vi "DCAM_show_preview_update_camera.vi"() -> ()   [LabVIEW 2015]
panel:
  out "S Start Trig Mode":dbl
  out "S Binning":dbl
  in  "Start Trigger Mode":u32(ring)=1 items=["Internal"=1, "External Edge"=2, "External Level"=4, "Software"=32, "Fast Repetition"=64, "TDI"=128, "Trigger Start"=512, "Sync Readout"=1024]
  in  "Binning":u16(ring) items=["1x1"=1, "2x2"=2, "4x4"=4]
  out "S Vert Offset":i32
  out "S Horiz Offset":i32
  in  "Vertical Offset":i32 min=0 max=0 step=4
  in  "Horizontal Offset":i32 min=0 max=0 step=4
  in  "Scan Mode":dbl min=1.0 max=2.0 step=1.0
  out "S Scan Mode":dbl min=1.0 max=2.0 step=1.0
  in  "Exposure":dbl min=0.0010036691729323308 max=10.000004210526315 step=1e-08
  out "S Exposure":dbl
  out "S Vert Width":i32
  out "S Horiz Width":i32
  in  "Vertical Width":i32 min=4 max=2048 step=4
  in  "Horizontal Width":i32 min=4 max=2048 step=4
  out "error out":errorcluster
  out "DCAM Ver.":string
  out "Library Ver.":string
  out "Firmware":string
  out "Camera ID":string
  out "Model":string
  out "Timeseries Base Filename":string
  out "Timeseries Save Path":path
  in  "Start Button":bool
  out "Image":u16[][](graph)
  in  "Stop":bool
  out "Frames Recorded":i32
  in  "Frames":i32=100
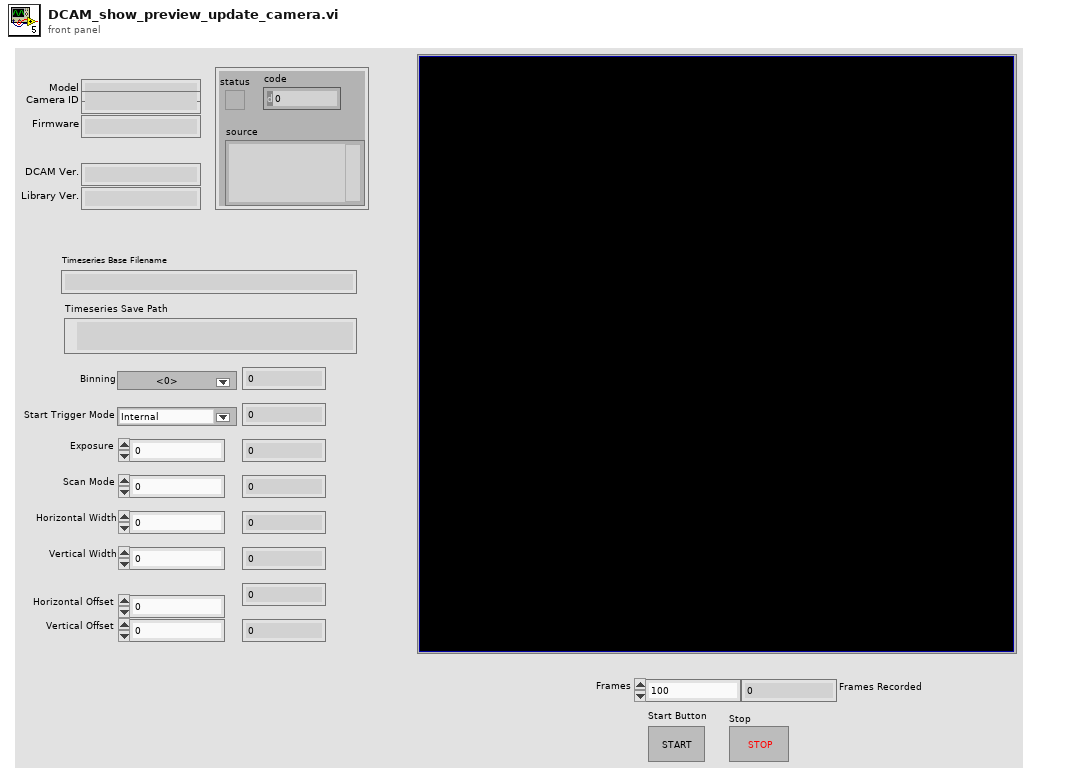
[diagram p1: front panel]
types:
  T1 = cluster{"Capture Library":string, "DCAM-API":string}
  T2 = cluster{"Model":string, "Camera ID":string, "Firmware":string}
  T3 = cluster{"Value":i32, "Minimum":i32, "Maximum":i32, "Increment":i32}
  T4 = cluster{"height":u32, "width":u32, "datatype":u32}
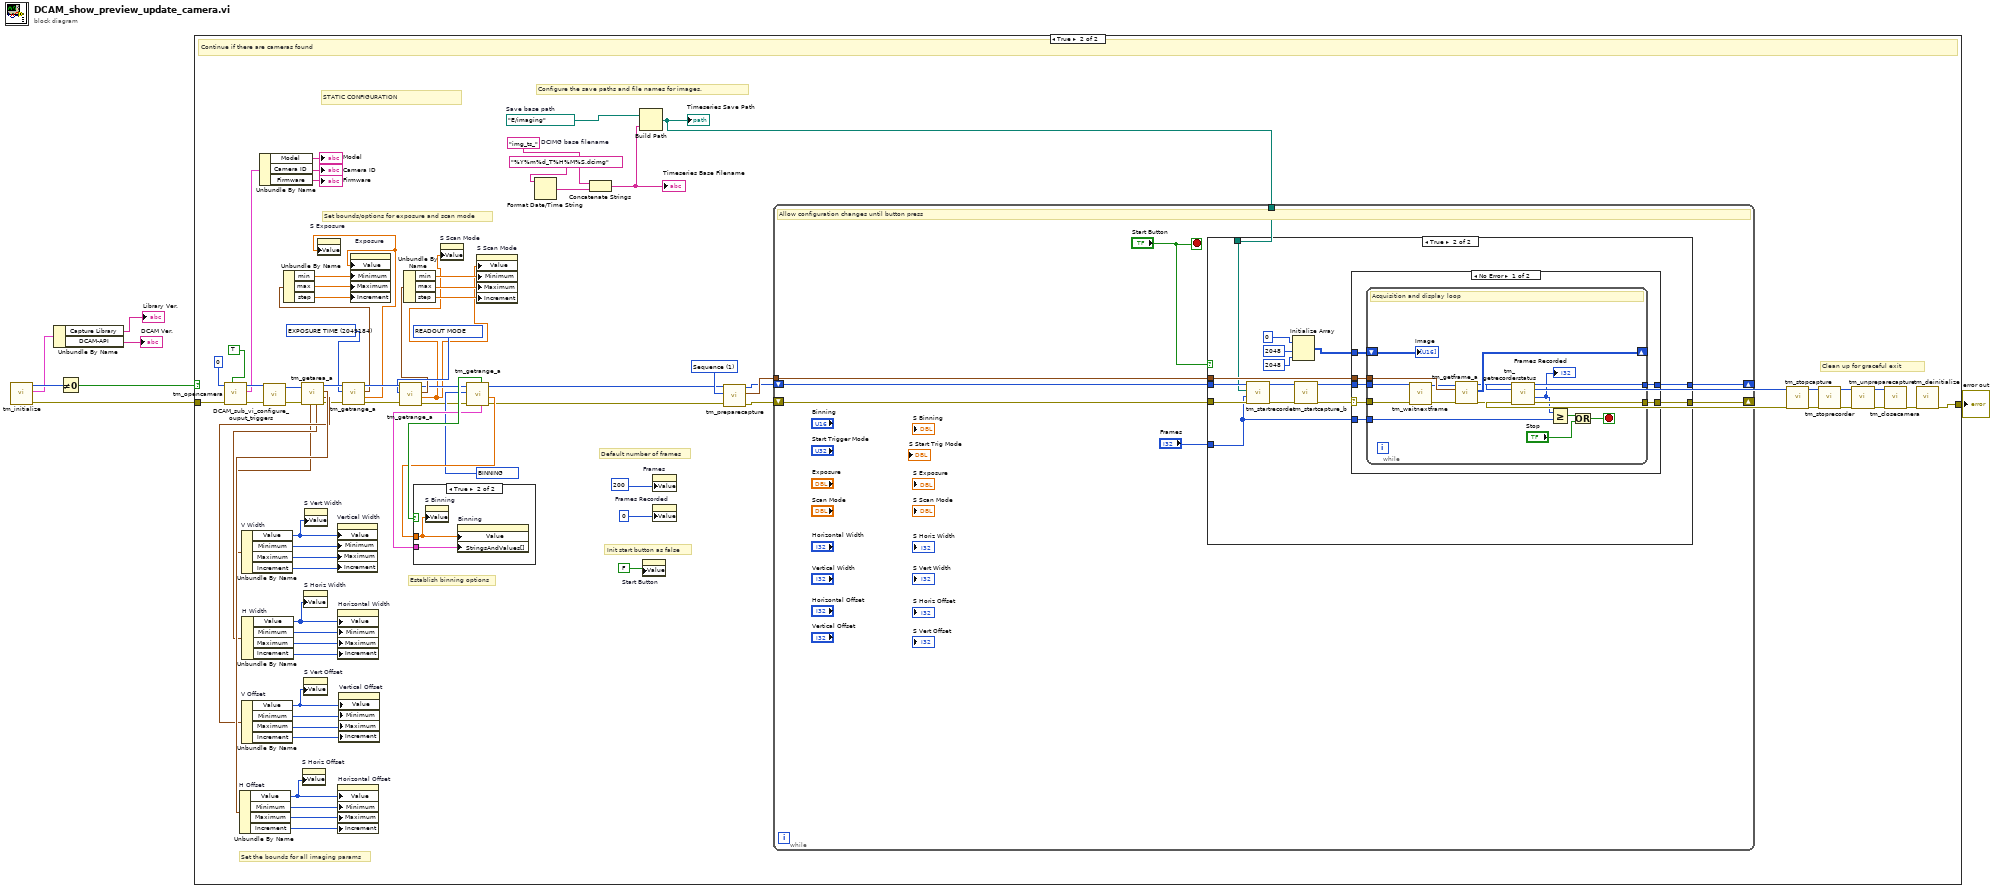
[diagram p0: block diagram]
diagram:
  n1 = call <userlib>:"tm_initialize.vi"() -> ("error out"=w2:errorcluster, "Version Info"=w5:T1, "Number Of Cameras"=w7:u32)  [unwired: 8 in, 1 out]
  n2 = Unbundle By Name(w5) -> ("Capture Library"=→"Library Ver.":string, "DCAM-API"=→"DCAM Ver.":string)
  n3 = Not Equal To 0?(x=w7) -> (x != 0?=w6:bool)
  n4 = case shown="True" w6 {
    tunnel: w2 -> [w8 w85]
    tunnel: [w8 w74] -> w1
    frame False {
    }
    frame True {
      w15 = u32 4215968 items=["BINNING"=4215968, "BITS PER CHANNEL"=4342976, "ACTIVE VIEW INDEX"=4343136, "CCD MODE"=4212384, "SENSOR MODE"=4212128, "READOUT MODE"=4211872, "EXPOSURE TIME"=2049184, "CONTRAST GAIN"=3163312, "CONTRAST OFFSET"=3163328, "LIGHT MODE"=2114720, "SENSITIVITY"=2114992, "WHITE BALANCE"=3163568, "PHOTON IMAGING MODE"=2115200, "HIGH DYNAMIC RANGE MODE"=3163360, "TRIGGER SOURCE"=1066144, "TRIGGER ACTIVE"=1066160, "TRIGGER MODE"=1066400, "TRIGGER POLARITY"=1066416, "TRIGGER GLOBAL EXPOSURE"=2049680, "FIRST TRIGGER BEHAVIOR"=2049696, "TRIGGER TIMES"=1066448, "OUTPUT TRIGGER POLARITY"=1852592, "OUTPUT TRIGGER DELAY"=1852624, "OUTPUT TRIGGER PERIOD"=1852640, "TEMPERATURE"=2115232, "TEMPERATURE TARGET"=2115264, "SENSOR COOLER FAN"=2115296, "MECHANICAL SHUTTER"=2115488, "BACK FOCUS POSITION"=8422304, "FRAMEBUNDLE MODE"=4346784, "FRAMEBUNDLE NUMBER"=4346800, "LINEBUNDLE HEIGHT"=4212192, "TRIGGER CONNECTOR"=1066432, "IMAGE PIXEL TYPE"=4343296, "OUTPUT TRIGGER KIND"=1852656, "READOUT DIRECTION"=4211904, "CHANNEL SYNC"=1852352] ("Parameter")
      w21 = u32 4211872 items=["BINNING"=4215968, "BITS PER CHANNEL"=4342976, "ACTIVE VIEW INDEX"=4343136, "CCD MODE"=4212384, "SENSOR MODE"=4212128, "READOUT MODE"=4211872, "EXPOSURE TIME"=2049184, "CONTRAST GAIN"=3163312, "CONTRAST OFFSET"=3163328, "LIGHT MODE"=2114720, "SENSITIVITY"=2114992, "WHITE BALANCE"=3163568, "PHOTON IMAGING MODE"=2115200, "HIGH DYNAMIC RANGE MODE"=3163360, "TRIGGER SOURCE"=1066144, "TRIGGER ACTIVE"=1066160, "TRIGGER MODE"=1066400, "TRIGGER POLARITY"=1066416, "TRIGGER GLOBAL EXPOSURE"=2049680, "FIRST TRIGGER BEHAVIOR"=2049696, "TRIGGER TIMES"=1066448, "OUTPUT TRIGGER POLARITY"=1852592, "OUTPUT TRIGGER DELAY"=1852624, "OUTPUT TRIGGER PERIOD"=1852640, "TEMPERATURE"=2115232, "TEMPERATURE TARGET"=2115264, "SENSOR COOLER FAN"=2115296, "MECHANICAL SHUTTER"=2115488, "BACK FOCUS POSITION"=8422304, "FRAMEBUNDLE MODE"=4346784, "FRAMEBUNDLE NUMBER"=4346800, "LINEBUNDLE HEIGHT"=4212192, "TRIGGER CONNECTOR"=1066432, "IMAGE PIXEL TYPE"=4343296, "OUTPUT TRIGGER KIND"=1852656, "READOUT DIRECTION"=4211904, "CHANNEL SYNC"=1852352] ("Parameter")
      w26 = u32 2049184 items=["BINNING"=4215968, "BITS PER CHANNEL"=4342976, "ACTIVE VIEW INDEX"=4343136, "CCD MODE"=4212384, "SENSOR MODE"=4212128, "READOUT MODE"=4211872, "EXPOSURE TIME"=2049184, "CONTRAST GAIN"=3163312, "CONTRAST OFFSET"=3163328, "LIGHT MODE"=2114720, "SENSITIVITY"=2114992, "WHITE BALANCE"=3163568, "PHOTON IMAGING MODE"=2115200, "HIGH DYNAMIC RANGE MODE"=3163360, "TRIGGER SOURCE"=1066144, "TRIGGER ACTIVE"=1066160, "TRIGGER MODE"=1066400, "TRIGGER POLARITY"=1066416, "TRIGGER GLOBAL EXPOSURE"=2049680, "FIRST TRIGGER BEHAVIOR"=2049696, "TRIGGER TIMES"=1066448, "OUTPUT TRIGGER POLARITY"=1852592, "OUTPUT TRIGGER DELAY"=1852624, "OUTPUT TRIGGER PERIOD"=1852640, "TEMPERATURE"=2115232, "TEMPERATURE TARGET"=2115264, "SENSOR COOLER FAN"=2115296, "MECHANICAL SHUTTER"=2115488, "BACK FOCUS POSITION"=8422304, "FRAMEBUNDLE MODE"=4346784, "FRAMEBUNDLE NUMBER"=4346800, "LINEBUNDLE HEIGHT"=4212192, "TRIGGER CONNECTOR"=1066432, "IMAGE PIXEL TYPE"=4343296, "OUTPUT TRIGGER KIND"=1852656, "READOUT DIRECTION"=4211904, "CHANNEL SYNC"=1852352] ("Parameter")
      w73 = 1 items=["Snap", "Sequence"] ("Capture mode")
      w59 = "img_ts_"  # DCIMG base filename
      w62 = path "E:/imaging"  # Save base path
      # "STATIC CONFIGURATION"
      # "Set bounds/options for exposure and scan mode"
      # "Establish binning options"
      # "Set the bounds for all imaging params"
      # "Init start button as false"
      # "Clean up for graceful exit"
      # "Default number of frames"
      # "Configure the save paths and file names for images."
      # "Continue if there are cameras found"
      n5 = call <userlib>:"tm_opencamera.vi"("Force Open"=TRUE, "error in (no error)"=w85, "Camera Index"=0) -> ("error out"=w82:errorcluster, "Camera Details"=w78:T2, "Handle out"=w83:u32)  [unwired: 6 in]
      n6 = Unbundle By Name(w78) -> ("Model"=→"Model":string, "Camera ID"=→"Camera ID":string, "Firmware"=→"Firmware":string)
      n7 = call "DCAM_sub_vi_configure_ouput_triggers.vi"("error in (no error)"=w82, "Handle in"=w83) -> ("error out"=w41:errorcluster, "Handle out"=w42:u32)  [unwired: 2 in]
      n8 = call <userlib>:"tm_getarea_a.vi"("error in (no error)"=w41, "Handle in"=w42) -> ("error out"=w34:errorcluster, "V Offset"=w37:T3, "H Offset"=w40:T3, "Handle out"=w39:u32, "H Width"=w36:T3, "V Width"=w35:T3)  [unwired: 4 in]
      n9 = Unbundle By Name "H Offset"(w40) -> ("Value"=w32:i32, "Minimum"=w45:i32, "Maximum"=w44:i32, "Increment"=w43:i32)
      n10 = Unbundle By Name "V Width"(w35) -> ("Value"=w29:i32, "Minimum"=w54:i32, "Maximum"=w53:i32, "Increment"=w52:i32)
      n11 = Unbundle By Name "V Offset"(w37) -> ("Value"=w31:i32, "Minimum"=w48:i32, "Maximum"=w47:i32, "Increment"=w46:i32)
      n12 = Unbundle By Name "H Width"(w36) -> ("Value"=w30:i32, "Minimum"=w51:i32, "Maximum"=w50:i32, "Increment"=w49:i32)
      n13 = property on="S Horiz Offset" class="DigNum (strict)"("Value"=w32) -> ()  [unwired: 2 in, 2 out]
      n14 = property on="S Horiz Width" class="DigNum (strict)"("Value"=w30) -> ()  [unwired: 2 in, 2 out]
      n15 = property on="S Vert Offset" class="DigNum (strict)"("Value"=w31) -> ()  [unwired: 2 in, 2 out]
      n16 = property on="S Vert Width" class="DigNum (strict)"("Value"=w29) -> ()  [unwired: 2 in, 2 out]
      n17 = property on="Vertical Width" class="DigNum (strict)"("Value"=w29, "Minimum"=w54, "Maximum"=w53, "Increment"=w52) -> ()  [unwired: 2 in, 2 out]
      n18 = property on="Horizontal Width" class="DigNum (strict)"("Value"=w30, "Minimum"=w51, "Maximum"=w50, "Increment"=w49) -> ()  [unwired: 2 in, 2 out]
      n19 = property on="Horizontal Offset" class="DigNum (strict)"("Value"=w32, "Minimum"=w45, "Maximum"=w44, "Increment"=w43) -> ()  [unwired: 2 in, 2 out]
      n20 = property on="Vertical Offset" class="DigNum (strict)"("Value"=w31, "Minimum"=w48, "Maximum"=w47, "Increment"=w46) -> ()  [unwired: 2 in, 2 out]
      n21 = call <userlib>:"tm_getrange_a.vi"("error in (no error)"=w34, "Parameter"=w26, "Handle in"=w39) -> ("error out"=w33:errorcluster, "default"=w10:dbl, "Range"=w25:cluster{"min":dbl, "max":dbl, "step":dbl}, "Handle out"=w38:u32)  [unwired: 2 in, 3 out]
      n22 = Unbundle By Name(w25) -> ("min"=w24:dbl, "max"=w27:dbl, "step"=w28:dbl)
      n23 = property on="S Exposure" class="DigNum (strict)"("Value"=w10) -> ()  [unwired: 2 in, 2 out]
      n24 = property on="Exposure" class="DigNum (strict)"("Value"=w10, "Minimum"=w24, "Maximum"=w27, "Increment"=w28) -> ()  [unwired: 2 in, 2 out]
      n25 = call <userlib>:"tm_getrange_a.vi"("error in (no error)"=w33, "Parameter"=w21, "Handle in"=w38) -> ("error out"=w13:errorcluster, "default"=w9:dbl, "Range"=w20:cluster{"min":dbl, "max":dbl, "step":dbl}, "Handle out"=w14:u32)  [unwired: 2 in, 3 out]
      n26 = Unbundle By Name(w20) -> ("min"=w19:dbl, "max"=w22:dbl, "step"=w23:dbl)
      n27 = property on="S Scan Mode" class="DigNum (strict)"("Value"=w9) -> ()  [unwired: 2 in, 2 out]
      n28 = call <userlib>:"tm_getrange_a.vi"("error in (no error)"=w13, "Parameter"=w15, "Handle in"=w14) -> ("error out"=w11:errorcluster, "default"=w17:dbl, "Handle out"=w12:u32, "Value Names"=w16:cluster{"Name":string, "Value":dbl}[], "Writable"=w18:bool)  [unwired: 2 in, 2 out]
      n29 = case shown="True" w18 {
        tunnel: w16 -> [_ w88]
        tunnel: w17 -> [_ w87]
        frame False {
        }
        frame True {
          n30 = property on="S Binning" class="DigNum (strict)"("Value"=w87) -> ()  [unwired: 2 in, 2 out]
          n31 = property on="Binning" class="Ring (strict)"("Value"=w87, "StringsAndValues[]"=w88) -> ()  [unwired: 2 in, 2 out]
        }
      }
      n32 = property on="S Scan Mode" class="DigNum (strict)"("Value"=w9, "Minimum"=w19, "Maximum"=w22, "Increment"=w23) -> ()  [unwired: 2 in, 2 out]
      n33 = Format Date/Time String(time format string (%c)="%Y%m%d_T%H%M%S.dcimg" ("name or relative path")) -> (date/time string=w60:string)  [unwired: 2 in]
      n34 = Concatenate Strings(w59, w60) -> (w57:string)
      "Timeseries Base Filename" <- w57
      n35 = Build Path(base path=w62, name or relative path=w57) -> (appended path=w58:path)
      "Timeseries Save Path" <- w58
      n36 = property on="Start Button" class="Bool (strict)"("Value"=FALSE) -> ()  [unwired: 2 in, 2 out]
      n37 = property on="Frames" class="DigNum (strict)"("Value"=200) -> ()  [unwired: 2 in, 2 out]
      n38 = property on="Frames Recorded" class="DigNum (strict)"("Value"=0) -> ()  [unwired: 2 in, 2 out]
      n39 = call <userlib>:"tm_preparecapture.vi"("error in (no error)"=w11, "Capture mode"=w73, "Handle in"=w12) -> ("error out"=w70:errorcluster, "Buffer Info"=w72:T4, "Handle out"=w71:u32)  [unwired: 5 in, 1 out]
      n40 = while {
        tunnel: w72 -> [w96]
        tunnel: w58 -> [w91]
        shift-right: [w93] -> w68
        shift-left: w71 -> [w95]
        shift-right: [w92] -> w67
        shift-left: w70 -> [w94]
        stop <- "Start Button" stop-if-true
        # "Allow configuration changes until button press"
        n41 = case shown="True" "Start Button" {
          tunnel: w96 -> [_ w113]
          tunnel: w95 -> [w98 w105]
          tunnel: w94 -> [w97 w104]
          tunnel: [w98 w103] -> w93
          tunnel: [w97 w102] -> w92
          tunnel: "Frames" -> [_ w101]
          tunnel: w91 -> [_ w99]
          frame False {
          }
          frame True {
            n42 = call <userlib>:"tm_startrecorder.vi"("error in (no error)"=w104, "frames"=w101, "File"=w99, "Handle in"=w105) -> ("error out"=w107:errorcluster, "Handle out"=w106:u32)  [unwired: 6 in]
            n43 = Initialize Array(u16 0 ("element"), 2048 ("dimension size"), 2048 ("dimension size")) -> (w108:u16[][])
            n44 = call <userlib>:"tm_startcapture_b.vi"("error in (no error)"=w107, "Handle in"=w106) -> ("error out"=w100:errorcluster, "Handle out"=w112:u32)  [unwired: 8 in]
            n45 = case shown="No Error" w100 {
              selector: w100 -> [w114 w138]
              tunnel: w113 -> [w120 _]
              tunnel: w112 -> [w119 w137]
              tunnel: w108 -> [w118 _]
              tunnel: [w117 w137] -> w103
              tunnel: [w116 w138] -> w102
              tunnel: w101 -> [w115 _]
              frame No Error {
                n46 = while {
                  tunnel: w120 -> [w136]
                  tunnel: w119 -> [w135]
                  tunnel: w114 -> [w132]
                  shift-right: [w130] -> _
                  shift-left: w118 -> [w131]
                  tunnel: [w127] -> w117
                  tunnel: [w126] -> w116
                  tunnel: w115 -> [w121]
                  stop <- w124 stop-if-true
                  # "Acquisition and display loop"
                  n47 = call <userlib>:"tm_waitnextframe.vi"("error in (no error)"=w132, "Handle in"=w135) -> ("error out"=w133:errorcluster, "Handle out"=w134:u32)  [unwired: 6 in, 2 out]
                  n48 = call <userlib>:"tm_getframe_a.vi"("error in (no error)"=w133, "Buffer Info"=w136, "Handle in"=w134) -> ("error out"=w129:errorcluster, "Data 16"=w130:u16[][], "Handle out"=w128:u32)  [unwired: 4 in, 2 out]
                  n49 = call <userlib>:"tm_getrecorderstatus.vi"("error in (no error)"=w129, "Handle"=w128) -> ("error out"=w126:errorcluster, "Count"=w122:i32, "Handle"=w127:u32)  [unwired: 6 in, 1 out]
                  "Frames Recorded" <- w122
                  n50 = Greater Or Equal?(x=w122, y=w121) -> (x >= y?=w123:bool)
                  n51 = Or(x=w123, y="Stop") -> (x .or. y?=w124:bool)
                  "Image" <- w131
                }
              }
              frame Error {
              }
            }
          }
        }
      }
      n52 = call <userlib>:"tm_stopcapture.vi"("error in (no error)"=w67, "Handle in"=w68) -> ("error out"=w63:errorcluster, "Handle out"=w64:u32)  [unwired: 8 in]
      n53 = call <userlib>:"tm_stoprecorder.vi"("error in (no error)"=w63, "Handle in"=w64) -> ("error out"=w65:errorcluster, "Handle out"=w66:u32)  [unwired: 8 in]
      n54 = call <userlib>:"tm_unpreparecapture.vi"("error in (no error)"=w65, "Handle in"=w66) -> ("error out"=w77:errorcluster, "Handle out"=w76:u32)  [unwired: 8 in]
      n55 = call <userlib>:"tm_closecamera.vi"("error in (no error)"=w77, "Handle in"=w76) -> ("error out"=w75:errorcluster)  [unwired: 9 in]
      n56 = call <userlib>:"tm_deinitialize.vi"("error in (no error)"=w75) -> ("error out"=w74:errorcluster)  [unwired: 10 in]
    }
  }
  "error out" <- w1
